vi "6Decembre2016.vi"() -> ()   [LabVIEW 2014]
panel:
  out "charMoins":string
  out "LettreMoins":i32
  out "Partie 2":string
  out "Partie 1":string
  out "charPlus":string
  out "LettrePlus":i32
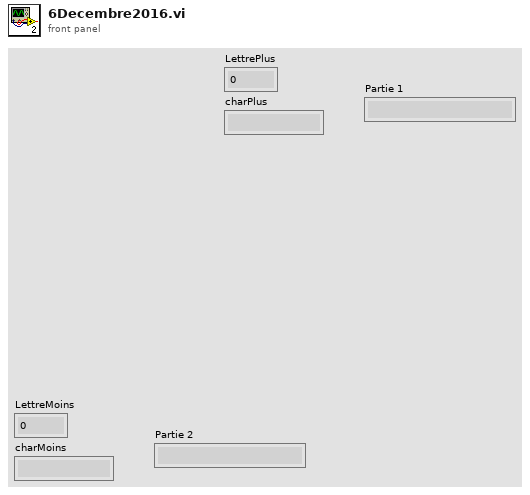
[diagram p1: front panel]
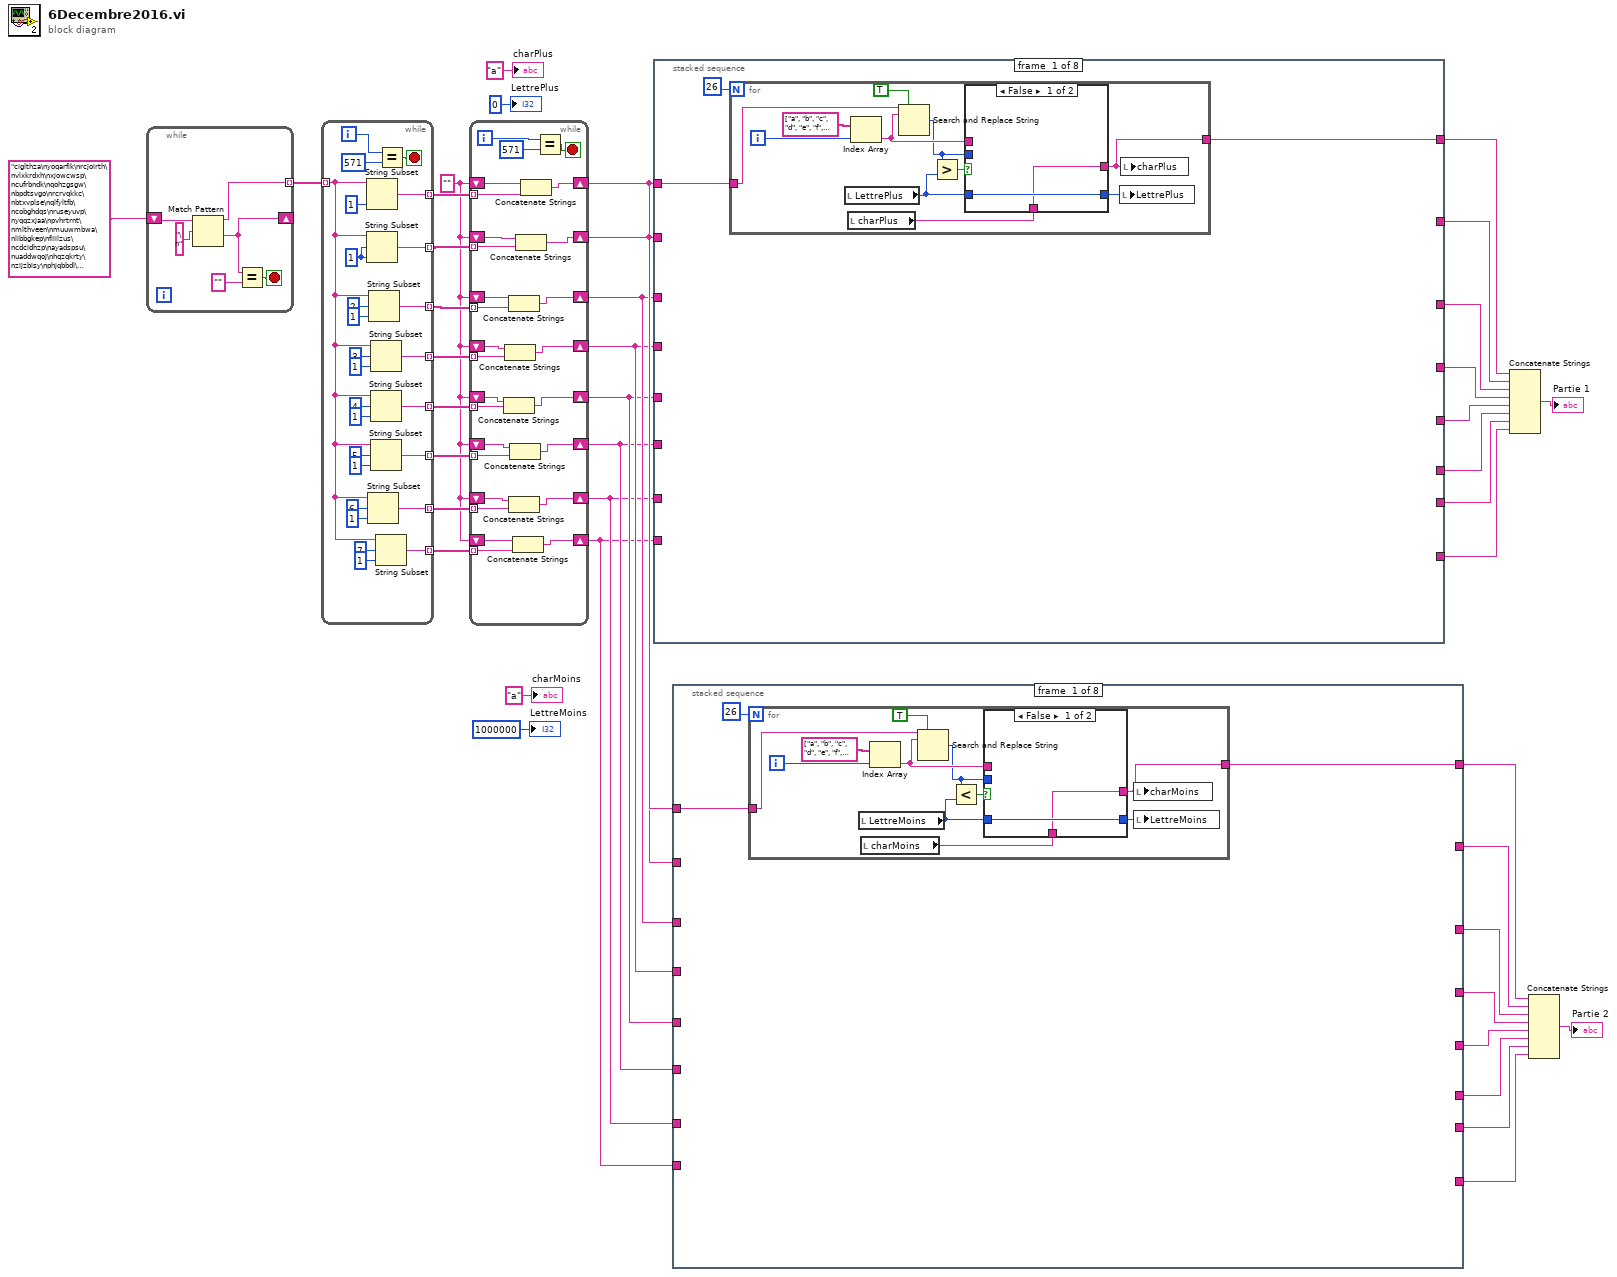
[diagram p0: block diagram]
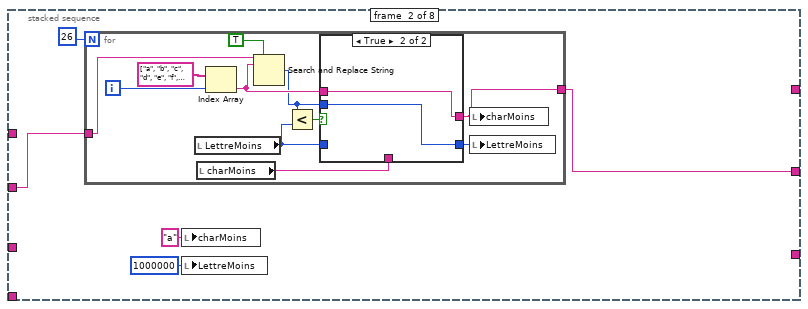
[diagram p3: hidden frame]
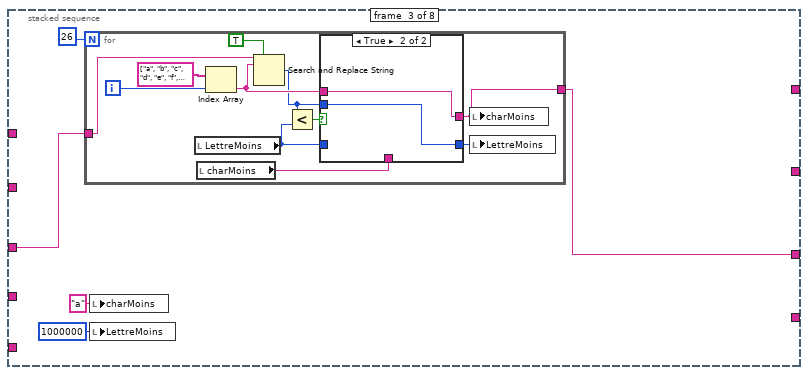
[diagram p5: hidden frame]
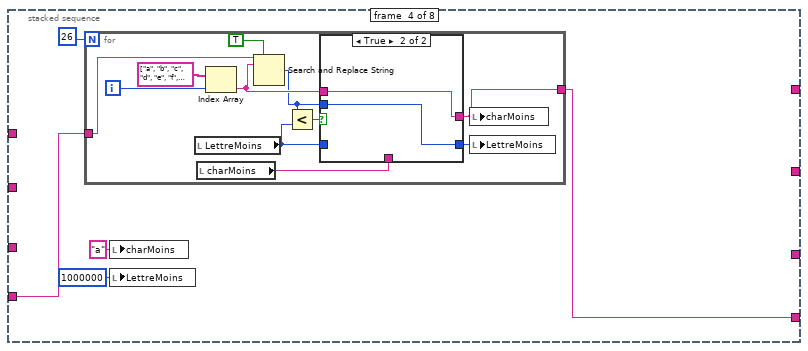
[diagram p7: hidden frame]
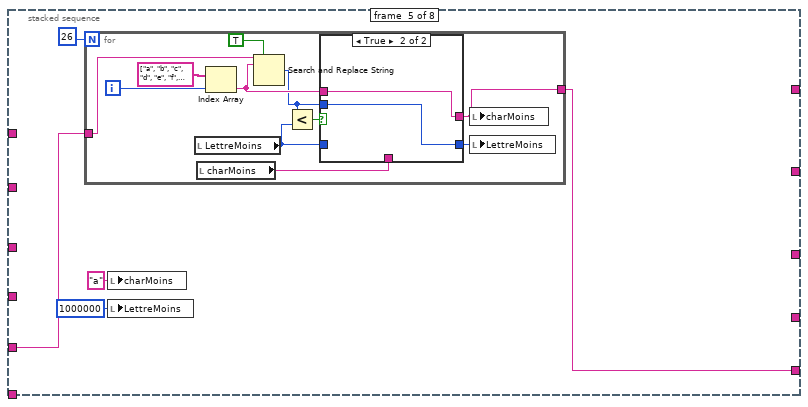
[diagram p9: hidden frame]
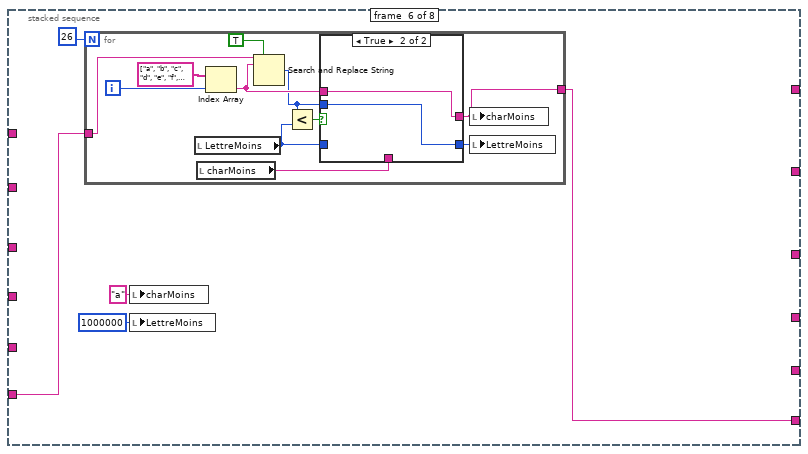
[diagram p11: hidden frame]
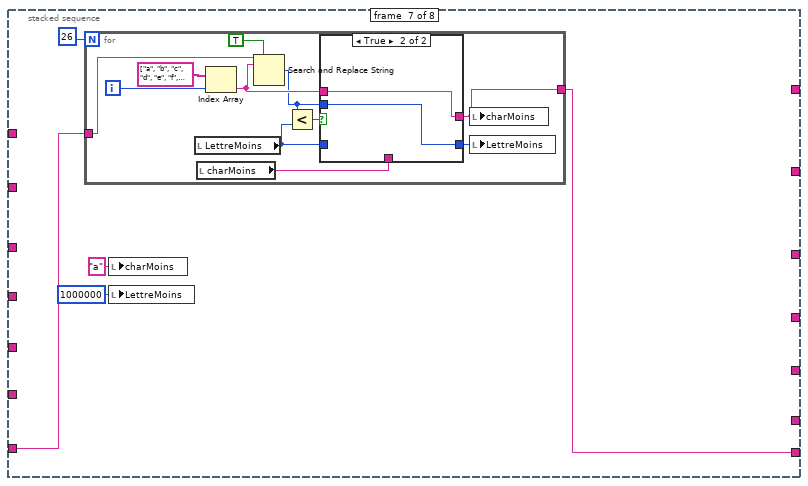
[diagram p13: hidden frame]
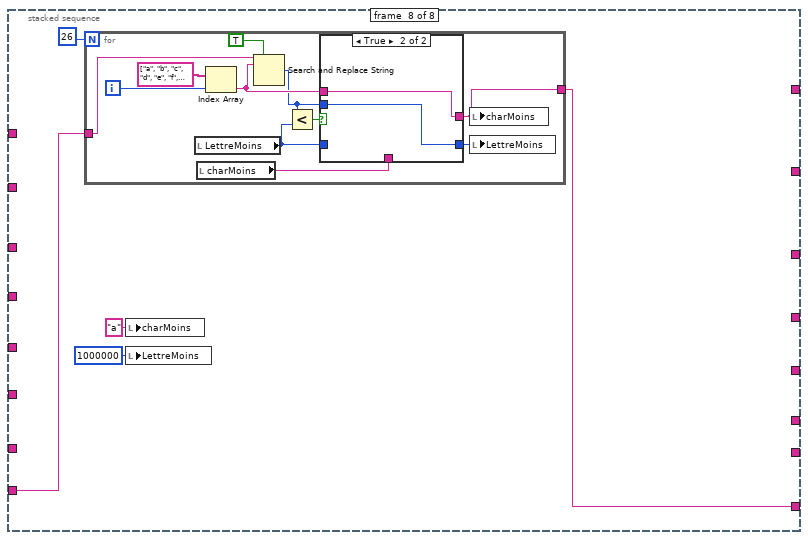
[diagram p15: hidden frame]
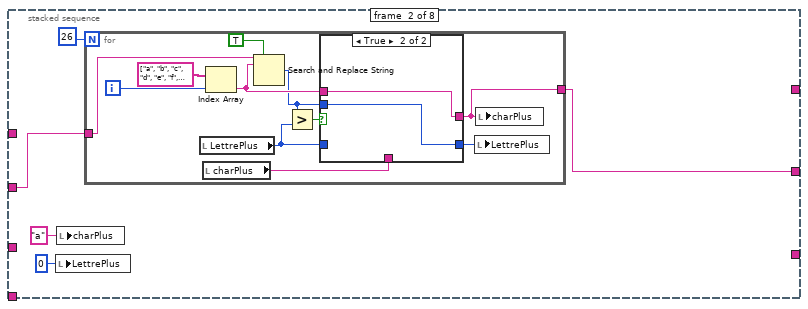
[diagram p18: hidden frame]
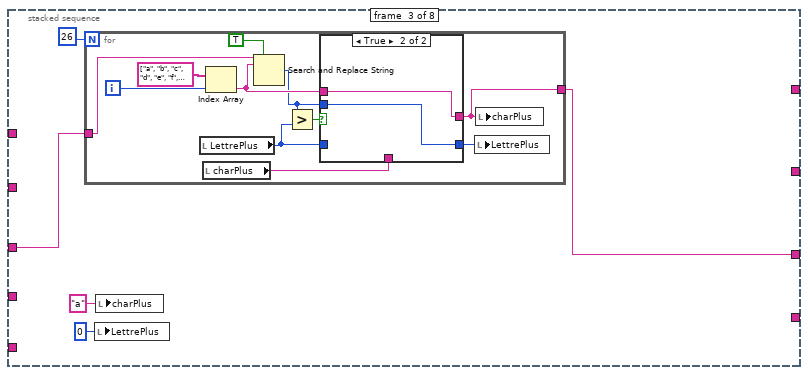
[diagram p20: hidden frame]
diagram:
  w31 = ""
  n1 = while {
    shift-right: [w44] -> _
    shift-left: "ciglthza\nyoqarfik\nrcjoirth\nvlxkrdxh\nxjowcwsp\ncufrbndk\nqohzgsgw\nbpdtsvgo\nrcrvqkkc\nbtxvplse\nqlfyltfb\ncobghdqs\nruseyuvp\nyqqzxjaa\npvhrtrnt\nmlthveen\nmuuwmbwa\nlibbgkep\nfiiilzus\ncdcidhzp\nayadspsu\nuaddwqoj\nhqzqkrty\nzijzbisy\nphjqbbdl\nmpqggfew\nasflznfc\nzmjrsxpj\nhsuvqnqf\ncfnafevn\npyotikpr\nzbpyuuwm\nkobzhfjl\nixzhdvlt\nkaocobts\nzvibydrv\napmgptcz\nxwlmhenu\nkxejeclq\nhxoouxor\nrlytjgev\nqaftppcw\nsozxfiaf\nsudsdedx\ndfkcuabm\nqztpvgtk\nbkifclzk\nesoukwnn\nzrhtjxfe\noqgzifhj\nafksfxxd\njkdlwctq\ndasojhxp\nrrztjdvp\ndvmkvwya\nbsclbdrg\nndemfsnm\nqbjidkwk\njfaknqge\nncrjolpa\neavqddsb\nfvkpfxvq\nowpgmxxq\ncaqrcygs\npzxjqtkx\nrfidiweg\nrgtptf..." -> [w47]
    tunnel: [w46] -> w40 mode=indexing
    stop <- w45 stop-if-true
    n2 = Match Pattern(string=w47, regular expression="\n") -> (before substring=w46:string, after substring=w44:string)  [unwired: 1 in, 2 out]
    n3 = Equal?(x=w44, y="") -> (x = y?=w45:bool)
  }
  n4 = while {
    tunnel: w40 -> [w56] mode=indexing
    tunnel: [w55] -> w33 mode=indexing
    tunnel: [w54] -> w32 mode=indexing
    tunnel: [w53] -> w34 mode=indexing
    tunnel: [w52] -> w35 mode=indexing
    tunnel: [w51] -> w36 mode=indexing
    tunnel: [w50] -> w37 mode=indexing
    tunnel: [w49] -> w38 mode=indexing
    tunnel: [w48] -> w39 mode=indexing
    i -> [w72]
    stop <- w73 stop-if-true
    w69 = 1 ("length (rest)")
    n5 = String Subset(string=w56, length (rest)=1 ("length (rest)")) -> (substring=w48:string)  [unwired: 1 in]
    n6 = String Subset(string=w56, offset (0)=w69, length (rest)=w69) -> (substring=w49:string)
    n7 = String Subset(string=w56, offset (0)=6, length (rest)=1 ("length (rest)")) -> (substring=w55:string)
    n8 = String Subset(string=w56, offset (0)=2, length (rest)=1 ("length (rest)")) -> (substring=w50:string)
    n9 = String Subset(string=w56, offset (0)=3, length (rest)=1 ("length (rest)")) -> (substring=w51:string)
    n10 = String Subset(string=w56, offset (0)=4, length (rest)=1 ("length (rest)")) -> (substring=w52:string)
    n11 = String Subset(string=w56, offset (0)=5, length (rest)=1 ("length (rest)")) -> (substring=w53:string)
    n12 = String Subset(string=w56, offset (0)=7, length (rest)=1 ("length (rest)")) -> (substring=w54:string)
    n13 = Equal?(x=w72, y=571) -> (x = y?=w73:bool)
  }
  n14 = while {
    tunnel: w39 -> [w100] mode=indexing
    shift-right: [w98] -> w8
    shift-left: w31 -> [w99]
    tunnel: w38 -> [w97] mode=indexing
    tunnel: w37 -> [w93] mode=indexing
    shift-right: [w91] -> w7
    shift-left: w31 -> [w92]
    shift-right: [w90] -> w6
    shift-left: w31 -> [w74]
    tunnel: w36 -> [w89] mode=indexing
    tunnel: w35 -> [w88] mode=indexing
    tunnel: w34 -> [w87] mode=indexing
    tunnel: w33 -> [w86] mode=indexing
    tunnel: w32 -> [w85] mode=indexing
    shift-right: [w75] -> w5
    shift-left: w31 -> [w83]
    shift-right: [w76] -> w4
    shift-left: w31 -> [w82]
    shift-right: [w77] -> w3
    shift-left: w31 -> [w81]
    shift-right: [w78] -> w2
    shift-left: w31 -> [w80]
    shift-right: [w79] -> w1
    shift-left: w31 -> [w84]
    i -> [w94]
    stop <- w95 stop-if-true
    n15 = Concatenate Strings(w82, w88) -> (w76:string)
    n16 = Concatenate Strings(w83, w89) -> (w75:string)
    n17 = Concatenate Strings(w74, w93) -> (w90:string)
    n18 = Concatenate Strings(w80, w86) -> (w78:string)
    n19 = Concatenate Strings(w81, w87) -> (w77:string)
    n20 = Concatenate Strings(w84, w85) -> (w79:string)
    n21 = Concatenate Strings(w92, w97) -> (w91:string)
    n22 = Concatenate Strings(w99, w100) -> (w98:string)
    n23 = Equal?(x=w94, y=571) -> (x = y?=w95:bool)
  }
  n24 = stacked-sequence {
    tunnel: w8 -> [w102 _ _ _ _ _ _ _]
    tunnel: [w101 _ _ _ _ _ _ _] -> w30
    tunnel: w7 -> [_ w122 _ _ _ _ _ _]
    tunnel: [_ w121 _ _ _ _ _ _] -> w29
    tunnel: w6 -> [_ _ w142 _ _ _ _ _]
    tunnel: [_ _ w141 _ _ _ _ _] -> w28
    tunnel: w5 -> [_ _ _ w162 _ _ _ _]
    tunnel: [_ _ _ w161 _ _ _ _] -> w27
    tunnel: w4 -> [_ _ _ _ w182 _ _ _]
    tunnel: [_ _ _ _ w181 _ _ _] -> w26
    tunnel: w3 -> [_ _ _ _ _ w202 _ _]
    tunnel: [_ _ _ _ _ w201 _ _] -> w25
    tunnel: w2 -> [_ _ _ _ _ _ w222 _]
    tunnel: [_ _ _ _ _ _ w221 _] -> w24
    tunnel: w1 -> [_ _ _ _ _ _ _ w242]
    tunnel: [_ _ _ _ _ _ _ w241] -> w23
    frame #0 {
      n25 = for {
        N: 26 -> [_]
        tunnel: w102 -> [w111]
        tunnel: [w104] -> w101
        i -> [w113]
        n26 = local read "LettrePlus"() -> (w109:i32)
        n27 = local read "charPlus"() -> (w107:string)
        n28 = Index Array(array=string[] ["a", "b", "c", "d", "e", "f", "g", "h", "i", "j", "k", "l", "m", "n", "o", "p", "q", "r", "s", "t", "u", "v", "w", "x", "y", "z"], index=w113) -> (element=w106:string)
        n29 = Search and Replace String(replace all?=TRUE ("replace all? (F)"), input string=w111, search string=w106) -> (number of replacements=w105:i32)  [unwired: 5 in, 3 out]
        n30 = Greater?(x=w105, y=w109) -> (0:w110:bool)
        n31 = case shown="False" w110 {
          tunnel: w109 -> [w116 _]
          tunnel: [w116 w117] -> w108
          tunnel: w107 -> [w115 _]
          tunnel: [w115 w118] -> w104
          tunnel: w106 -> [_ w118]
          tunnel: w105 -> [_ w117]
          frame False {
          }
          frame True {
          }
        }
        n32 = local write "LettrePlus"(w108) -> ()
        n33 = local write "charPlus"(w104) -> ()
      }
    }
    frame #1 {
      n34 = local write "LettrePlus"(0 ("LettrePlus")) -> ()
      n35 = local write "charPlus"("a" ("charPlus")) -> ()
      n36 = for {
        N: 26 -> [_]
        tunnel: w122 -> [w131]
        tunnel: [w124] -> w121
        i -> [w133]
        n37 = local read "LettrePlus"() -> (w129:i32)
        n38 = local read "charPlus"() -> (w127:string)
        n39 = Index Array(array=string[] ["a", "b", "c", "d", "e", "f", "g", "h", "i", "j", "k", "l", "m", "n", "o", "p", "q", "r", "s", "t", "u", "v", "w", "x", "y", "z"], index=w133) -> (element=w126:string)
        n40 = Search and Replace String(replace all?=TRUE ("replace all? (F)"), input string=w131, search string=w126) -> (number of replacements=w125:i32)  [unwired: 5 in, 3 out]
        n41 = Greater?(x=w125, y=w129) -> (0:w130:bool)
        n42 = case shown="True" w130 {
          tunnel: w129 -> [w136 _]
          tunnel: [w136 w137] -> w128
          tunnel: w127 -> [w135 _]
          tunnel: [w135 w138] -> w124
          tunnel: w126 -> [_ w138]
          tunnel: w125 -> [_ w137]
          frame False {
          }
          frame True {
          }
        }
        n43 = local write "LettrePlus"(w128) -> ()
        n44 = local write "charPlus"(w124) -> ()
      }
    }
    frame #2 {
      n45 = for {
        N: 26 -> [_]
        tunnel: w142 -> [w151]
        tunnel: [w144] -> w141
        i -> [w153]
        n46 = local read "LettrePlus"() -> (w149:i32)
        n47 = local read "charPlus"() -> (w147:string)
        n48 = Index Array(array=string[] ["a", "b", "c", "d", "e", "f", "g", "h", "i", "j", "k", "l", "m", "n", "o", "p", "q", "r", "s", "t", "u", "v", "w", "x", "y", "z"], index=w153) -> (element=w146:string)
        n49 = Search and Replace String(replace all?=TRUE ("replace all? (F)"), input string=w151, search string=w146) -> (number of replacements=w145:i32)  [unwired: 5 in, 3 out]
        n50 = Greater?(x=w145, y=w149) -> (0:w150:bool)
        n51 = case shown="True" w150 {
          tunnel: w149 -> [w156 _]
          tunnel: [w156 w157] -> w148
          tunnel: w147 -> [w155 _]
          tunnel: [w155 w158] -> w144
          tunnel: w146 -> [_ w158]
          tunnel: w145 -> [_ w157]
          frame False {
          }
          frame True {
          }
        }
        n52 = local write "LettrePlus"(w148) -> ()
        n53 = local write "charPlus"(w144) -> ()
      }
      n54 = local write "LettrePlus"(0 ("LettrePlus")) -> ()
      n55 = local write "charPlus"("a" ("charPlus")) -> ()
    }
    frame #3 {
      n56 = for {
        N: 26 -> [_]
        tunnel: w162 -> [w171]
        tunnel: [w164] -> w161
        i -> [w173]
        n57 = local read "LettrePlus"() -> (w169:i32)
        n58 = local read "charPlus"() -> (w167:string)
        n59 = Index Array(array=string[] ["a", "b", "c", "d", "e", "f", "g", "h", "i", "j", "k", "l", "m", "n", "o", "p", "q", "r", "s", "t", "u", "v", "w", "x", "y", "z"], index=w173) -> (element=w166:string)
        n60 = Search and Replace String(replace all?=TRUE ("replace all? (F)"), input string=w171, search string=w166) -> (number of replacements=w165:i32)  [unwired: 5 in, 3 out]
        n61 = Greater?(x=w165, y=w169) -> (0:w170:bool)
        n62 = case shown="True" w170 {
          tunnel: w169 -> [w176 _]
          tunnel: [w176 w177] -> w168
          tunnel: w167 -> [w175 _]
          tunnel: [w175 w178] -> w164
          tunnel: w166 -> [_ w178]
          tunnel: w165 -> [_ w177]
          frame False {
          }
          frame True {
          }
        }
        n63 = local write "LettrePlus"(w168) -> ()
        n64 = local write "charPlus"(w164) -> ()
      }
      n65 = local write "LettrePlus"(0 ("LettrePlus")) -> ()
      n66 = local write "charPlus"("a" ("charPlus")) -> ()
    }
    frame #4 {
      n67 = for {
        N: 26 -> [_]
        tunnel: w182 -> [w191]
        tunnel: [w184] -> w181
        i -> [w193]
        n68 = local read "LettrePlus"() -> (w189:i32)
        n69 = local read "charPlus"() -> (w187:string)
        n70 = Index Array(array=string[] ["a", "b", "c", "d", "e", "f", "g", "h", "i", "j", "k", "l", "m", "n", "o", "p", "q", "r", "s", "t", "u", "v", "w", "x", "y", "z"], index=w193) -> (element=w186:string)
        n71 = Search and Replace String(replace all?=TRUE ("replace all? (F)"), input string=w191, search string=w186) -> (number of replacements=w185:i32)  [unwired: 5 in, 3 out]
        n72 = Greater?(x=w185, y=w189) -> (0:w190:bool)
        n73 = case shown="True" w190 {
          tunnel: w189 -> [w196 _]
          tunnel: [w196 w197] -> w188
          tunnel: w187 -> [w195 _]
          tunnel: [w195 w198] -> w184
          tunnel: w186 -> [_ w198]
          tunnel: w185 -> [_ w197]
          frame False {
          }
          frame True {
          }
        }
        n74 = local write "LettrePlus"(w188) -> ()
        n75 = local write "charPlus"(w184) -> ()
      }
      n76 = local write "LettrePlus"(0 ("LettrePlus")) -> ()
      n77 = local write "charPlus"("a" ("charPlus")) -> ()
    }
    frame #5 {
      n78 = for {
        N: 26 -> [_]
        tunnel: w202 -> [w211]
        tunnel: [w204] -> w201
        i -> [w213]
        n79 = local read "LettrePlus"() -> (w209:i32)
        n80 = local read "charPlus"() -> (w207:string)
        n81 = Index Array(array=string[] ["a", "b", "c", "d", "e", "f", "g", "h", "i", "j", "k", "l", "m", "n", "o", "p", "q", "r", "s", "t", "u", "v", "w", "x", "y", "z"], index=w213) -> (element=w206:string)
        n82 = Search and Replace String(replace all?=TRUE ("replace all? (F)"), input string=w211, search string=w206) -> (number of replacements=w205:i32)  [unwired: 5 in, 3 out]
        n83 = Greater?(x=w205, y=w209) -> (0:w210:bool)
        n84 = case shown="True" w210 {
          tunnel: w209 -> [w216 _]
          tunnel: [w216 w217] -> w208
          tunnel: w207 -> [w215 _]
          tunnel: [w215 w218] -> w204
          tunnel: w206 -> [_ w218]
          tunnel: w205 -> [_ w217]
          frame False {
          }
          frame True {
          }
        }
        n85 = local write "LettrePlus"(w208) -> ()
        n86 = local write "charPlus"(w204) -> ()
      }
      n87 = local write "LettrePlus"(0 ("LettrePlus")) -> ()
      n88 = local write "charPlus"("a" ("charPlus")) -> ()
    }
    frame #6 {
      n89 = for {
        N: 26 -> [_]
        tunnel: w222 -> [w231]
        tunnel: [w224] -> w221
        i -> [w233]
        n90 = local read "LettrePlus"() -> (w229:i32)
        n91 = local read "charPlus"() -> (w227:string)
        n92 = Index Array(array=string[] ["a", "b", "c", "d", "e", "f", "g", "h", "i", "j", "k", "l", "m", "n", "o", "p", "q", "r", "s", "t", "u", "v", "w", "x", "y", "z"], index=w233) -> (element=w226:string)
        n93 = Search and Replace String(replace all?=TRUE ("replace all? (F)"), input string=w231, search string=w226) -> (number of replacements=w225:i32)  [unwired: 5 in, 3 out]
        n94 = Greater?(x=w225, y=w229) -> (0:w230:bool)
        n95 = case shown="True" w230 {
          tunnel: w229 -> [w236 _]
          tunnel: [w236 w237] -> w228
          tunnel: w227 -> [w235 _]
          tunnel: [w235 w238] -> w224
          tunnel: w226 -> [_ w238]
          tunnel: w225 -> [_ w237]
          frame False {
          }
          frame True {
          }
        }
        n96 = local write "LettrePlus"(w228) -> ()
        n97 = local write "charPlus"(w224) -> ()
      }
      n98 = local write "LettrePlus"(0 ("LettrePlus")) -> ()
      n99 = local write "charPlus"("a" ("charPlus")) -> ()
    }
    frame #7 {
      n100 = for {
        N: 26 -> [_]
        tunnel: w242 -> [w251]
        tunnel: [w244] -> w241
        i -> [w253]
        n101 = local read "LettrePlus"() -> (w249:i32)
        n102 = local read "charPlus"() -> (w247:string)
        n103 = Index Array(array=string[] ["a", "b", "c", "d", "e", "f", "g", "h", "i", "j", "k", "l", "m", "n", "o", "p", "q", "r", "s", "t", "u", "v", "w", "x", "y", "z"], index=w253) -> (element=w246:string)
        n104 = Search and Replace String(replace all?=TRUE ("replace all? (F)"), input string=w251, search string=w246) -> (number of replacements=w245:i32)  [unwired: 5 in, 3 out]
        n105 = Greater?(x=w245, y=w249) -> (0:w250:bool)
        n106 = case shown="True" w250 {
          tunnel: w249 -> [w256 _]
          tunnel: [w256 w257] -> w248
          tunnel: w247 -> [w255 _]
          tunnel: [w255 w258] -> w244
          tunnel: w246 -> [_ w258]
          tunnel: w245 -> [_ w257]
          frame False {
          }
          frame True {
          }
        }
        n107 = local write "LettrePlus"(w248) -> ()
        n108 = local write "charPlus"(w244) -> ()
      }
      n109 = local write "LettrePlus"(0 ("LettrePlus")) -> ()
      n110 = local write "charPlus"("a" ("charPlus")) -> ()
    }
  }
  n111 = stacked-sequence {
    tunnel: w8 -> [w260 _ _ _ _ _ _ _]
    tunnel: [w259 _ _ _ _ _ _ _] -> w19
    tunnel: w7 -> [_ w280 _ _ _ _ _ _]
    tunnel: [_ w279 _ _ _ _ _ _] -> w18
    tunnel: w6 -> [_ _ w300 _ _ _ _ _]
    tunnel: [_ _ w299 _ _ _ _ _] -> w17
    tunnel: w5 -> [_ _ _ w320 _ _ _ _]
    tunnel: [_ _ _ w319 _ _ _ _] -> w16
    tunnel: w4 -> [_ _ _ _ w340 _ _ _]
    tunnel: [_ _ _ _ w339 _ _ _] -> w15
    tunnel: w3 -> [_ _ _ _ _ w360 _ _]
    tunnel: [_ _ _ _ _ w359 _ _] -> w14
    tunnel: w2 -> [_ _ _ _ _ _ w380 _]
    tunnel: [_ _ _ _ _ _ w379 _] -> w13
    tunnel: w1 -> [_ _ _ _ _ _ _ w400]
    tunnel: [_ _ _ _ _ _ _ w399] -> w12
    frame #0 {
      n112 = for {
        N: 26 -> [_]
        tunnel: w260 -> [w269]
        tunnel: [w262] -> w259
        i -> [w271]
        n113 = local read "LettreMoins"() -> (w267:i32)
        n114 = local read "charMoins"() -> (w265:string)
        n115 = Index Array(array=string[] ["a", "b", "c", "d", "e", "f", "g", "h", "i", "j", "k", "l", "m", "n", "o", "p", "q", "r", "s", "t", "u", "v", "w", "x", "y", "z"], index=w271) -> (element=w264:string)
        n116 = Search and Replace String(replace all?=TRUE ("replace all? (F)"), input string=w269, search string=w264) -> (number of replacements=w263:i32)  [unwired: 5 in, 3 out]
        n117 = Less?(x=w263, y=w267) -> (x < y?=w268:bool)
        n118 = case shown="False" w268 {
          tunnel: w267 -> [w274 _]
          tunnel: [w274 w275] -> w266
          tunnel: w265 -> [w273 _]
          tunnel: [w273 w276] -> w262
          tunnel: w264 -> [_ w276]
          tunnel: w263 -> [_ w275]
          frame False {
          }
          frame True {
          }
        }
        n119 = local write "charMoins"(w262) -> ()
        n120 = local write "LettreMoins"(w266) -> ()
      }
    }
    frame #1 {
      n121 = for {
        N: 26 -> [_]
        tunnel: w280 -> [w289]
        tunnel: [w282] -> w279
        i -> [w291]
        n122 = local read "LettreMoins"() -> (w287:i32)
        n123 = local read "charMoins"() -> (w285:string)
        n124 = Index Array(array=string[] ["a", "b", "c", "d", "e", "f", "g", "h", "i", "j", "k", "l", "m", "n", "o", "p", "q", "r", "s", "t", "u", "v", "w", "x", "y", "z"], index=w291) -> (element=w284:string)
        n125 = Search and Replace String(replace all?=TRUE ("replace all? (F)"), input string=w289, search string=w284) -> (number of replacements=w283:i32)  [unwired: 5 in, 3 out]
        n126 = Less?(x=w283, y=w287) -> (x < y?=w288:bool)
        n127 = case shown="True" w288 {
          tunnel: w287 -> [w294 _]
          tunnel: [w294 w295] -> w286
          tunnel: w285 -> [w293 _]
          tunnel: [w293 w296] -> w282
          tunnel: w284 -> [_ w296]
          tunnel: w283 -> [_ w295]
          frame False {
          }
          frame True {
          }
        }
        n128 = local write "charMoins"(w282) -> ()
        n129 = local write "LettreMoins"(w286) -> ()
      }
      n130 = local write "charMoins"("a" ("charPlus")) -> ()
      n131 = local write "LettreMoins"(1000000 ("LettrePlus")) -> ()
    }
    frame #2 {
      n132 = for {
        N: 26 -> [_]
        tunnel: w300 -> [w309]
        tunnel: [w302] -> w299
        i -> [w311]
        n133 = local read "LettreMoins"() -> (w307:i32)
        n134 = local read "charMoins"() -> (w305:string)
        n135 = Index Array(array=string[] ["a", "b", "c", "d", "e", "f", "g", "h", "i", "j", "k", "l", "m", "n", "o", "p", "q", "r", "s", "t", "u", "v", "w", "x", "y", "z"], index=w311) -> (element=w304:string)
        n136 = Search and Replace String(replace all?=TRUE ("replace all? (F)"), input string=w309, search string=w304) -> (number of replacements=w303:i32)  [unwired: 5 in, 3 out]
        n137 = Less?(x=w303, y=w307) -> (x < y?=w308:bool)
        n138 = case shown="True" w308 {
          tunnel: w307 -> [w314 _]
          tunnel: [w314 w315] -> w306
          tunnel: w305 -> [w313 _]
          tunnel: [w313 w316] -> w302
          tunnel: w304 -> [_ w316]
          tunnel: w303 -> [_ w315]
          frame False {
          }
          frame True {
          }
        }
        n139 = local write "charMoins"(w302) -> ()
        n140 = local write "LettreMoins"(w306) -> ()
      }
      n141 = local write "charMoins"("a" ("charPlus")) -> ()
      n142 = local write "LettreMoins"(1000000 ("LettrePlus")) -> ()
    }
    frame #3 {
      n143 = for {
        N: 26 -> [_]
        tunnel: w320 -> [w329]
        tunnel: [w322] -> w319
        i -> [w331]
        n144 = local read "LettreMoins"() -> (w327:i32)
        n145 = local read "charMoins"() -> (w325:string)
        n146 = Index Array(array=string[] ["a", "b", "c", "d", "e", "f", "g", "h", "i", "j", "k", "l", "m", "n", "o", "p", "q", "r", "s", "t", "u", "v", "w", "x", "y", "z"], index=w331) -> (element=w324:string)
        n147 = Search and Replace String(replace all?=TRUE ("replace all? (F)"), input string=w329, search string=w324) -> (number of replacements=w323:i32)  [unwired: 5 in, 3 out]
        n148 = Less?(x=w323, y=w327) -> (x < y?=w328:bool)
        n149 = case shown="True" w328 {
          tunnel: w327 -> [w334 _]
          tunnel: [w334 w335] -> w326
          tunnel: w325 -> [w333 _]
          tunnel: [w333 w336] -> w322
          tunnel: w324 -> [_ w336]
          tunnel: w323 -> [_ w335]
          frame False {
          }
          frame True {
          }
        }
        n150 = local write "charMoins"(w322) -> ()
        n151 = local write "LettreMoins"(w326) -> ()
      }
      n152 = local write "charMoins"("a" ("charPlus")) -> ()
      n153 = local write "LettreMoins"(1000000 ("LettrePlus")) -> ()
    }
    frame #4 {
      n154 = for {
        N: 26 -> [_]
        tunnel: w340 -> [w349]
        tunnel: [w342] -> w339
        i -> [w351]
        n155 = local read "LettreMoins"() -> (w347:i32)
        n156 = local read "charMoins"() -> (w345:string)
        n157 = Index Array(array=string[] ["a", "b", "c", "d", "e", "f", "g", "h", "i", "j", "k", "l", "m", "n", "o", "p", "q", "r", "s", "t", "u", "v", "w", "x", "y", "z"], index=w351) -> (element=w344:string)
        n158 = Search and Replace String(replace all?=TRUE ("replace all? (F)"), input string=w349, search string=w344) -> (number of replacements=w343:i32)  [unwired: 5 in, 3 out]
        n159 = Less?(x=w343, y=w347) -> (x < y?=w348:bool)
        n160 = case shown="True" w348 {
          tunnel: w347 -> [w354 _]
          tunnel: [w354 w355] -> w346
          tunnel: w345 -> [w353 _]
          tunnel: [w353 w356] -> w342
          tunnel: w344 -> [_ w356]
          tunnel: w343 -> [_ w355]
          frame False {
          }
          frame True {
          }
        }
        n161 = local write "charMoins"(w342) -> ()
        n162 = local write "LettreMoins"(w346) -> ()
      }
      n163 = local write "charMoins"("a" ("charPlus")) -> ()
      n164 = local write "LettreMoins"(1000000 ("LettrePlus")) -> ()
    }
    frame #5 {
      n165 = for {
        N: 26 -> [_]
        tunnel: w360 -> [w369]
        tunnel: [w362] -> w359
        i -> [w371]
        n166 = local read "LettreMoins"() -> (w367:i32)
        n167 = local read "charMoins"() -> (w365:string)
        n168 = Index Array(array=string[] ["a", "b", "c", "d", "e", "f", "g", "h", "i", "j", "k", "l", "m", "n", "o", "p", "q", "r", "s", "t", "u", "v", "w", "x", "y", "z"], index=w371) -> (element=w364:string)
        n169 = Search and Replace String(replace all?=TRUE ("replace all? (F)"), input string=w369, search string=w364) -> (number of replacements=w363:i32)  [unwired: 5 in, 3 out]
        n170 = Less?(x=w363, y=w367) -> (x < y?=w368:bool)
        n171 = case shown="True" w368 {
          tunnel: w367 -> [w374 _]
          tunnel: [w374 w375] -> w366
          tunnel: w365 -> [w373 _]
          tunnel: [w373 w376] -> w362
          tunnel: w364 -> [_ w376]
          tunnel: w363 -> [_ w375]
          frame False {
          }
          frame True {
          }
        }
        n172 = local write "charMoins"(w362) -> ()
        n173 = local write "LettreMoins"(w366) -> ()
      }
      n174 = local write "charMoins"("a" ("charPlus")) -> ()
      n175 = local write "LettreMoins"(1000000 ("LettrePlus")) -> ()
    }
    frame #6 {
      n176 = for {
        N: 26 -> [_]
        tunnel: w380 -> [w389]
        tunnel: [w382] -> w379
        i -> [w391]
        n177 = local read "LettreMoins"() -> (w387:i32)
        n178 = local read "charMoins"() -> (w385:string)
        n179 = Index Array(array=string[] ["a", "b", "c", "d", "e", "f", "g", "h", "i", "j", "k", "l", "m", "n", "o", "p", "q", "r", "s", "t", "u", "v", "w", "x", "y", "z"], index=w391) -> (element=w384:string)
        n180 = Search and Replace String(replace all?=TRUE ("replace all? (F)"), input string=w389, search string=w384) -> (number of replacements=w383:i32)  [unwired: 5 in, 3 out]
        n181 = Less?(x=w383, y=w387) -> (x < y?=w388:bool)
        n182 = case shown="True" w388 {
          tunnel: w387 -> [w394 _]
          tunnel: [w394 w395] -> w386
          tunnel: w385 -> [w393 _]
          tunnel: [w393 w396] -> w382
          tunnel: w384 -> [_ w396]
          tunnel: w383 -> [_ w395]
          frame False {
          }
          frame True {
          }
        }
        n183 = local write "charMoins"(w382) -> ()
        n184 = local write "LettreMoins"(w386) -> ()
      }
      n185 = local write "charMoins"("a" ("charPlus")) -> ()
      n186 = local write "LettreMoins"(1000000 ("LettrePlus")) -> ()
    }
    frame #7 {
      n187 = for {
        N: 26 -> [_]
        tunnel: w400 -> [w409]
        tunnel: [w402] -> w399
        i -> [w411]
        n188 = local read "LettreMoins"() -> (w407:i32)
        n189 = local read "charMoins"() -> (w405:string)
        n190 = Index Array(array=string[] ["a", "b", "c", "d", "e", "f", "g", "h", "i", "j", "k", "l", "m", "n", "o", "p", "q", "r", "s", "t", "u", "v", "w", "x", "y", "z"], index=w411) -> (element=w404:string)
        n191 = Search and Replace String(replace all?=TRUE ("replace all? (F)"), input string=w409, search string=w404) -> (number of replacements=w403:i32)  [unwired: 5 in, 3 out]
        n192 = Less?(x=w403, y=w407) -> (x < y?=w408:bool)
        n193 = case shown="True" w408 {
          tunnel: w407 -> [w414 _]
          tunnel: [w414 w415] -> w406
          tunnel: w405 -> [w413 _]
          tunnel: [w413 w416] -> w402
          tunnel: w404 -> [_ w416]
          tunnel: w403 -> [_ w415]
          frame False {
          }
          frame True {
          }
        }
        n194 = local write "charMoins"(w402) -> ()
        n195 = local write "LettreMoins"(w406) -> ()
      }
      n196 = local write "charMoins"("a" ("charPlus")) -> ()
      n197 = local write "LettreMoins"(1000000 ("LettrePlus")) -> ()
    }
  }
  n198 = Concatenate Strings(w30, w29, w28, w27, w26, w25, w24, w23) -> (→"Partie 1":string)
  n199 = Concatenate Strings(w19, w18, w17, w16, w15, w14, w13, w12) -> (→"Partie 2":string)
  "LettrePlus" <- 0 ("LettrePlus")
  "charPlus" <- "a" ("charPlus")
  "LettreMoins" <- 1000000 ("LettreMoins")
  "charMoins" <- "a" ("charMoins")
